vi "LVSgetAMtable.vi"(11 "Serial Port Select":refnum<visa-resource-name>="COM3") -> (0 "COM Error":bool, 1 "Min dB":dbl, 2 "Max dB":dbl, 3 "Waveform Graph":dbl[](graph), 4 "AM Freq Hz":dbl, 8 "Step Delay uS":dbl)   [LabVIEW 2017]
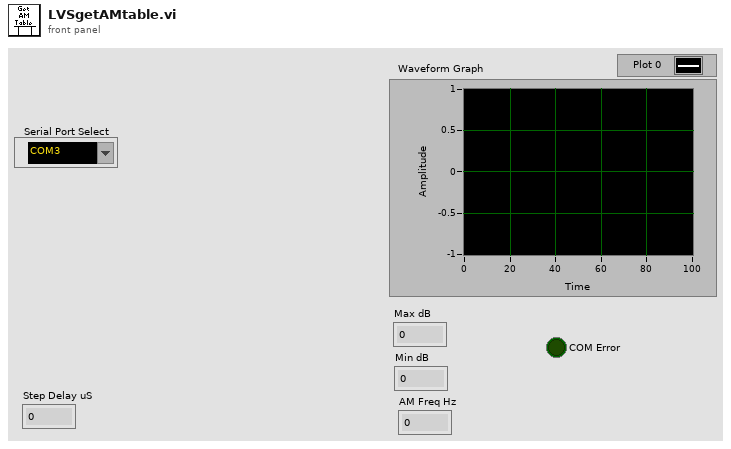
[diagram p1: front panel]
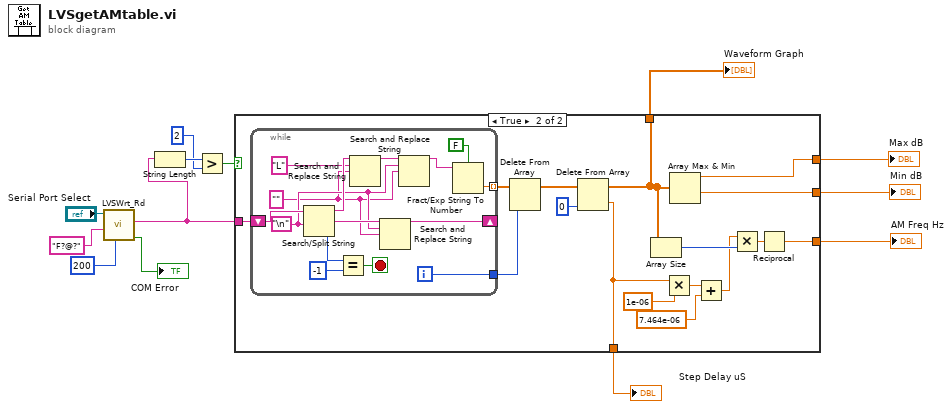
[diagram p0: block diagram]
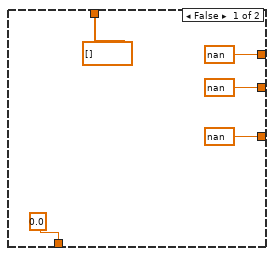
[diagram p2: hidden frame]
diagram:
  n1 = call "LVSWrt_Rd.vi"("delay"=u32 200, "WriteBuf"="F?@?" ("write buffer"), "COM Port"="Serial Port Select") -> ("ComError"=→"COM Error":bool, "string read"=w2:string)  [unwired: 7 in]
  n2 = String Length(string=w2) -> (length=w12:i32)
  n3 = Greater?(x=w12, y=2) -> (0:w13:bool)
  n4 = case shown="True" w13 {
    tunnel: w2 -> [_ w34]
    tunnel: [dbl[] [] w20] -> w10
    tunnel: [nan w26] -> w9
    tunnel: [nan w25] -> w8
    tunnel: [nan w24] -> w7
    tunnel: [0.0 w23] -> w6
    frame False {
    }
    frame True {
      n5 = while {
        shift-right: [w41] -> _
        shift-left: w34 -> [w47]
        tunnel: [w38] -> w33
        tunnel: [w36] -> w22 mode=indexing
        i -> [w38]
        stop <- w49 stop-if-true
        w40 = "\n"
        w39 = "" ("replace string (\"\")")
        n6 = Search/Split String(string=w47, search string/char (-)=w40) -> (substring before match=w46:string, match + rest of string=w42:string, offset of match=w43:i32)  [unwired: 1 in]
        n7 = Equal?(x=w43, y=-1) -> (x = y?=w49:bool)
        n8 = Search and Replace String(input string=w46, search string="L" ("format string"), replace string=w39) -> (result string=w44:string)  [unwired: 5 in, 3 out]
        n9 = Search and Replace String(input string=w42, search string=w40, replace string=w39) -> (result string=w41:string)  [unwired: 5 in, 3 out]
        n10 = Search and Replace String(input string=w44, search string=w40, replace string=w39) -> (result string=w37:string)  [unwired: 5 in, 3 out]
        n11 = Fract/Exp String To Number(use system decimal point (T)=FALSE, string=w37) -> (number=w36:dbl)  [unwired: 2 in, 1 out]
      }
      n12 = Delete From Array(array=w22, index=w33) -> (array with subset deleted=w21:dbl[])  [unwired: 1 in, 1 out]
      n13 = Delete From Array(array=w21, index=0) -> (deleted portion=w23:dbl, array with subset deleted=w20:dbl[])  [unwired: 1 in]
      n14 = Array Size(array=w20) -> (size(s)=w32:i32)
      n15 = Multiply(x=w23, y=1e-06) -> (x*y=w29:dbl)
      n16 = Array Max & Min(array=w20) -> (max value=w26:dbl, min value=w25:dbl)  [unwired: 2 out]
      n17 = Add(x=w29, y=7.464e-06 ("x")) -> (x+y=w27:dbl)
      n18 = Multiply(x=w27, y=w32) -> (x*y=w31:dbl)
      n19 = Reciprocal(x=w31) -> (1/x=w24:dbl)
    }
  }
  "Waveform Graph" <- w10
  "Step Delay uS" <- w6
  "AM Freq Hz" <- w7
  "Min dB" <- w8
  "Max dB" <- w9
